vi "SetAllTestStatus.vi"(10 "AllTestStatus":T1, 11 "Model in":refnum<class "Model.lvclass">) -> (3 "Model out":refnum<class "Model.lvclass">)   [LabVIEW 2016, in "Model.lvclass"]
uses:
  Model.lvclass
  Typedefs/AllTestStatus.ctl
  Typedefs/TestStatus.ctl
  Model.lvclass/Model.ctl
  Typedefs/FAMT Typedefs.lvlib
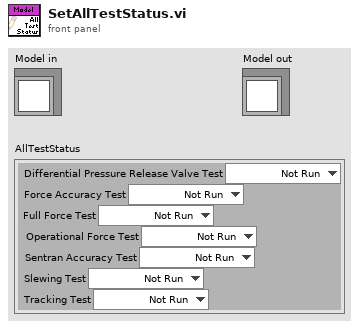
[diagram p1: front panel]
types:
  T1 = typedef "FAMT Typedefs.lvlib/AllTestStatus.ctl" = cluster{"Differential Pressure Release Valve Test":T2, "Force Accuracy Test":T2, "Full Force Test":T2, "Operational Force Test":T2, "Sentran Accuracy Test":T2, "Slewing Test":T2, "Tracking Test":T2}
  T2 = typedef "FAMT Typedefs.lvlib/TestStatus.ctl" = enum16{"Not Run", "Running", "Passed", "Failed"}
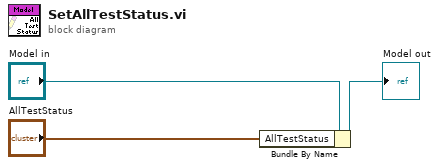
[diagram p0: block diagram]
diagram:
  n1 = Bundle By Name(cluster="Model in", "AllTestStatus"="AllTestStatus") -> (→"Model out":refnum<class "Model.lvclass">)
